vi "Test.vi"() -> ()   [LabVIEW 2019, in "Exaprom PDF.lvlib"]
uses:
  Exaprom PDF.lvlib
panel:
  out "String and format [ ]":T1(array[cluster])
  out "time (msec)":u32=27
  in  "String":string="A document can also contain images, tables, and columns. This part explains how iText implements these structures, and the examples demonstrate how they fit together."
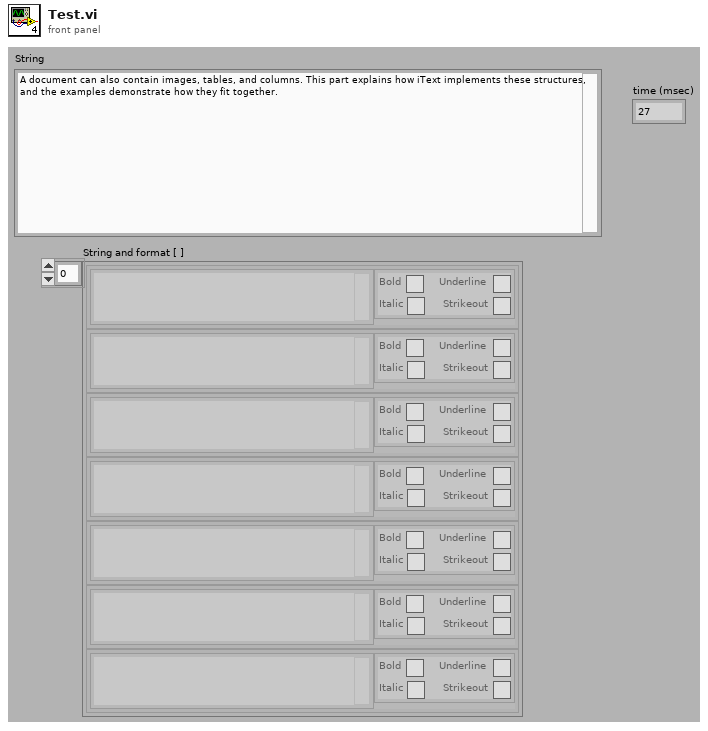
[diagram p1: front panel]
types:
  T1 = cluster{"string":string, "Style":cluster{"Bold":bool, "Italic":bool, "Underline":bool, "Strikeout":bool}}[]
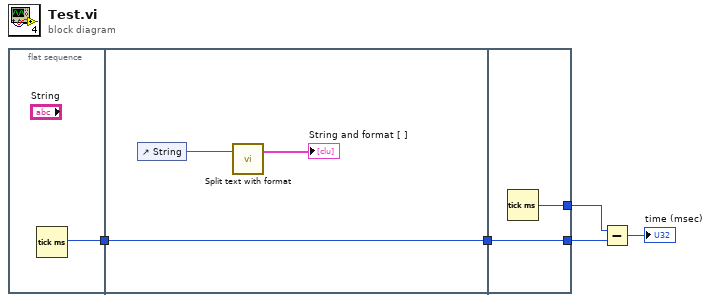
[diagram p0: block diagram]
diagram:
  n1 = flat-sequence {
    tunnel: [w6] -> w4
    tunnel: w4 -> [w8]
    tunnel: [w8] -> w3
    tunnel: [w11] -> w5
    tunnel: w3 -> [w10]
    tunnel: [w10] -> w2
    frame #0 {
      n2 = Tick Count (ms)() -> (millisecond timer value=w6:u32)
    }
    frame #1 {
      n3 = control-ref of="String"() -> (w9:refnum<vi>)
      n4 = call "Split text with format.vi"("Str Refnum"=w9) -> ("String and format [ ]"=→"String and format [ ]":T1)  [unwired: 1 in, 1 out]
    }
    frame #2 {
      n5 = Tick Count (ms)() -> (millisecond timer value=w11:u32)
    }
  }
  n6 = Subtract(x=w5, y=w2) -> (x-y=→"time (msec)":u32)
